vi "外观 2.vi"(0 "Data In":T8 caption="数据输入" {"数值" format="%04x"}, 2 "Display State In":T6 caption="显示状态输入", 3 "Container State":T7 caption="容器状态") -> (6 "Data Out":T8 caption="数据输出" {"数值" format="%04x"}, 7 "Display State Out":T6 caption="显示状态输出", 8 "Action":T5 caption="动作")   [LabVIEW 2016, in "CODMn调试控件V3.xctl"]
uses:
  <vilib>/_xctls/Container State.ctl
  <vilib>/_xctls/Action.ctl
  <vilib>/_xctls/XControlSupport.lvlib
panel:
  in  "模式":enum32{"测试模式", "流程模式"}(tab)
  in  "外设:":T1
  in  "加热:":bool caption="V2"
  in  "摄氏度":u16
  in  "量:":u16=5000
  in  "注射泵:":T2(radio)
  in  "偏心轮:":u16 caption="mL"
  in  "进样:":enum32{"未选择", "水样", "纯水", "标液", "零点", "加标回收"}(radio)
  in  "柱塞泵体积/等待时间":u16=5000
  in  "功能选择":enum32{"等待", "复位", "注入", "注出"}(radio)=enum."注入"
  out "选项卡控件":enum32{"选项卡 1", "选项卡 2"}(tab)
  in  "阀口选择":T3(radio)
  in  "其他":enum32{"未选择", "更新A值", "更新B值", "反滴定"}(radio)
  in  "反应杯温度控制:":u16
  in  "偏心轮抽取液体次数:":u16
  in  "外设":T4
  out "字符串":string="柱塞泵体积μL"
  # "uL"
  # "℃"
  # "次(0代表不动作)"
  # "℃(0代表不控温)"
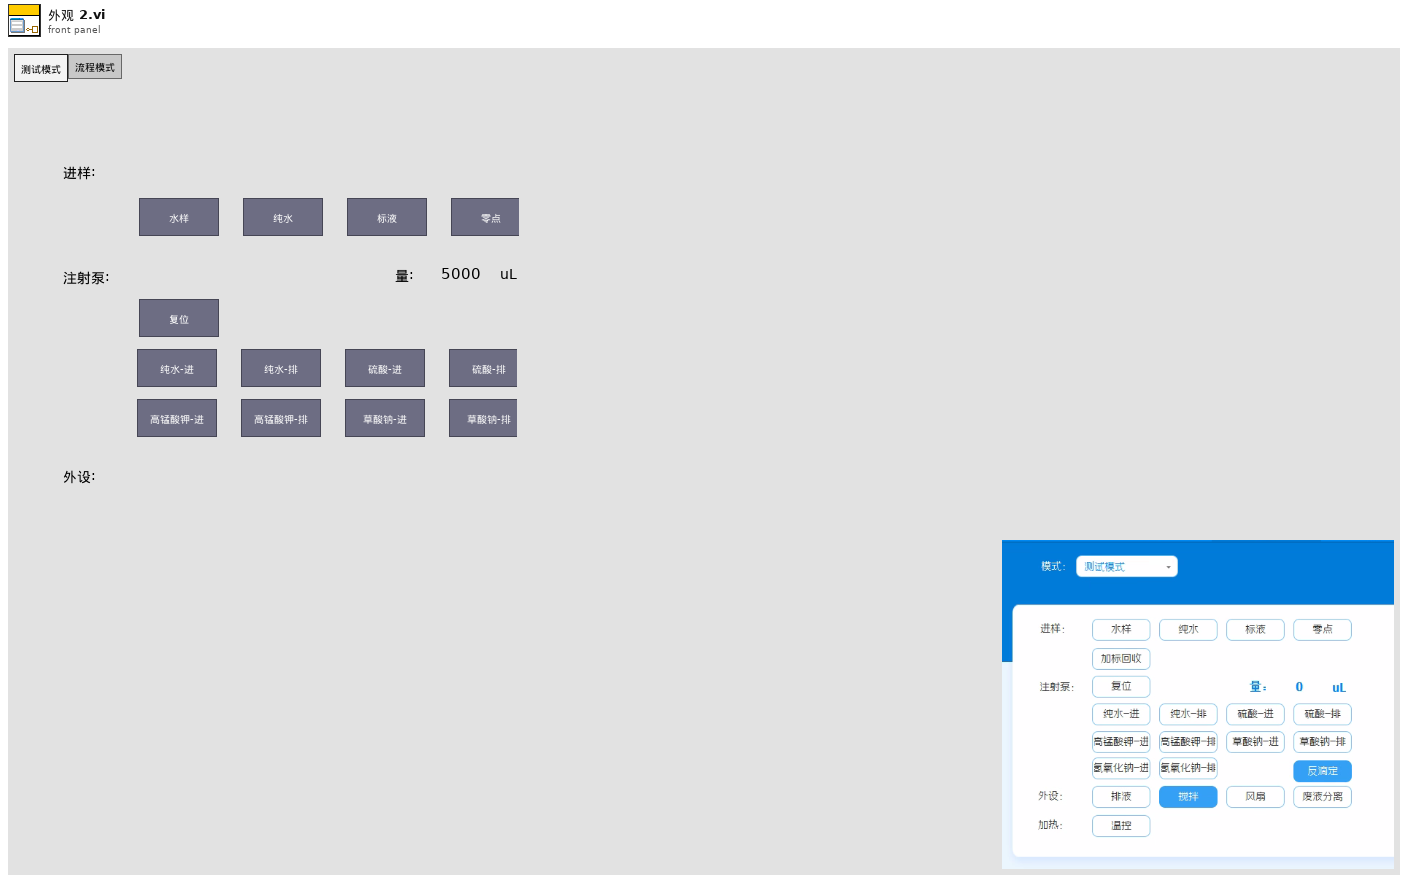
[diagram p1: front panel]
types:
  T1 = cluster{"排液":bool, "搅拌":bool, "风扇":bool, "废液分离":bool}
  T2 = enum32{"未选择", "纯水-进", "纯水-排", "硫酸-进", "硫酸-排", "复位", "高锰酸钾-进", "高锰酸钾-排", "草酸钠-进", "草酸钠-排", "氢氧化钠-进", "氢氧化钠-排", "反滴定"}
  T3 = enum32{"未选择", "V1", "V2", "V3", "V4", "V5", "V6", "V7", "V8", "V9", "V10", "V11", "V12"}
  T4 = cluster{"排液阀":bool, "搅拌":bool, "冷凝风扇":bool, "废液分离阀":bool, "电磁阀1":bool, "电磁阀2":bool, "电磁阀3":bool, "电磁阀4":bool}
  T5 = typedef "XControlSupport.lvlib/Action.ctl" = cluster{"Data Changed?":bool, "State Changed?":bool, "Action Name":string}
  T6 = typedef "CODMn调试控件V3.xctl/状态 2.ctl" = cluster{"Numeric":dbl}
  T7 = typedef "XControlSupport.lvlib/Container State.ctl" = cluster{"Indicator?":bool, "Run Mode?":bool, " Refnum":refnum<vi>}
  T8 = typedef "CODMn调试控件V3.xctl/数据 2.ctl" = cluster{"数值":u16[], "模式":enum32{"测试模式", "流程模式"}}
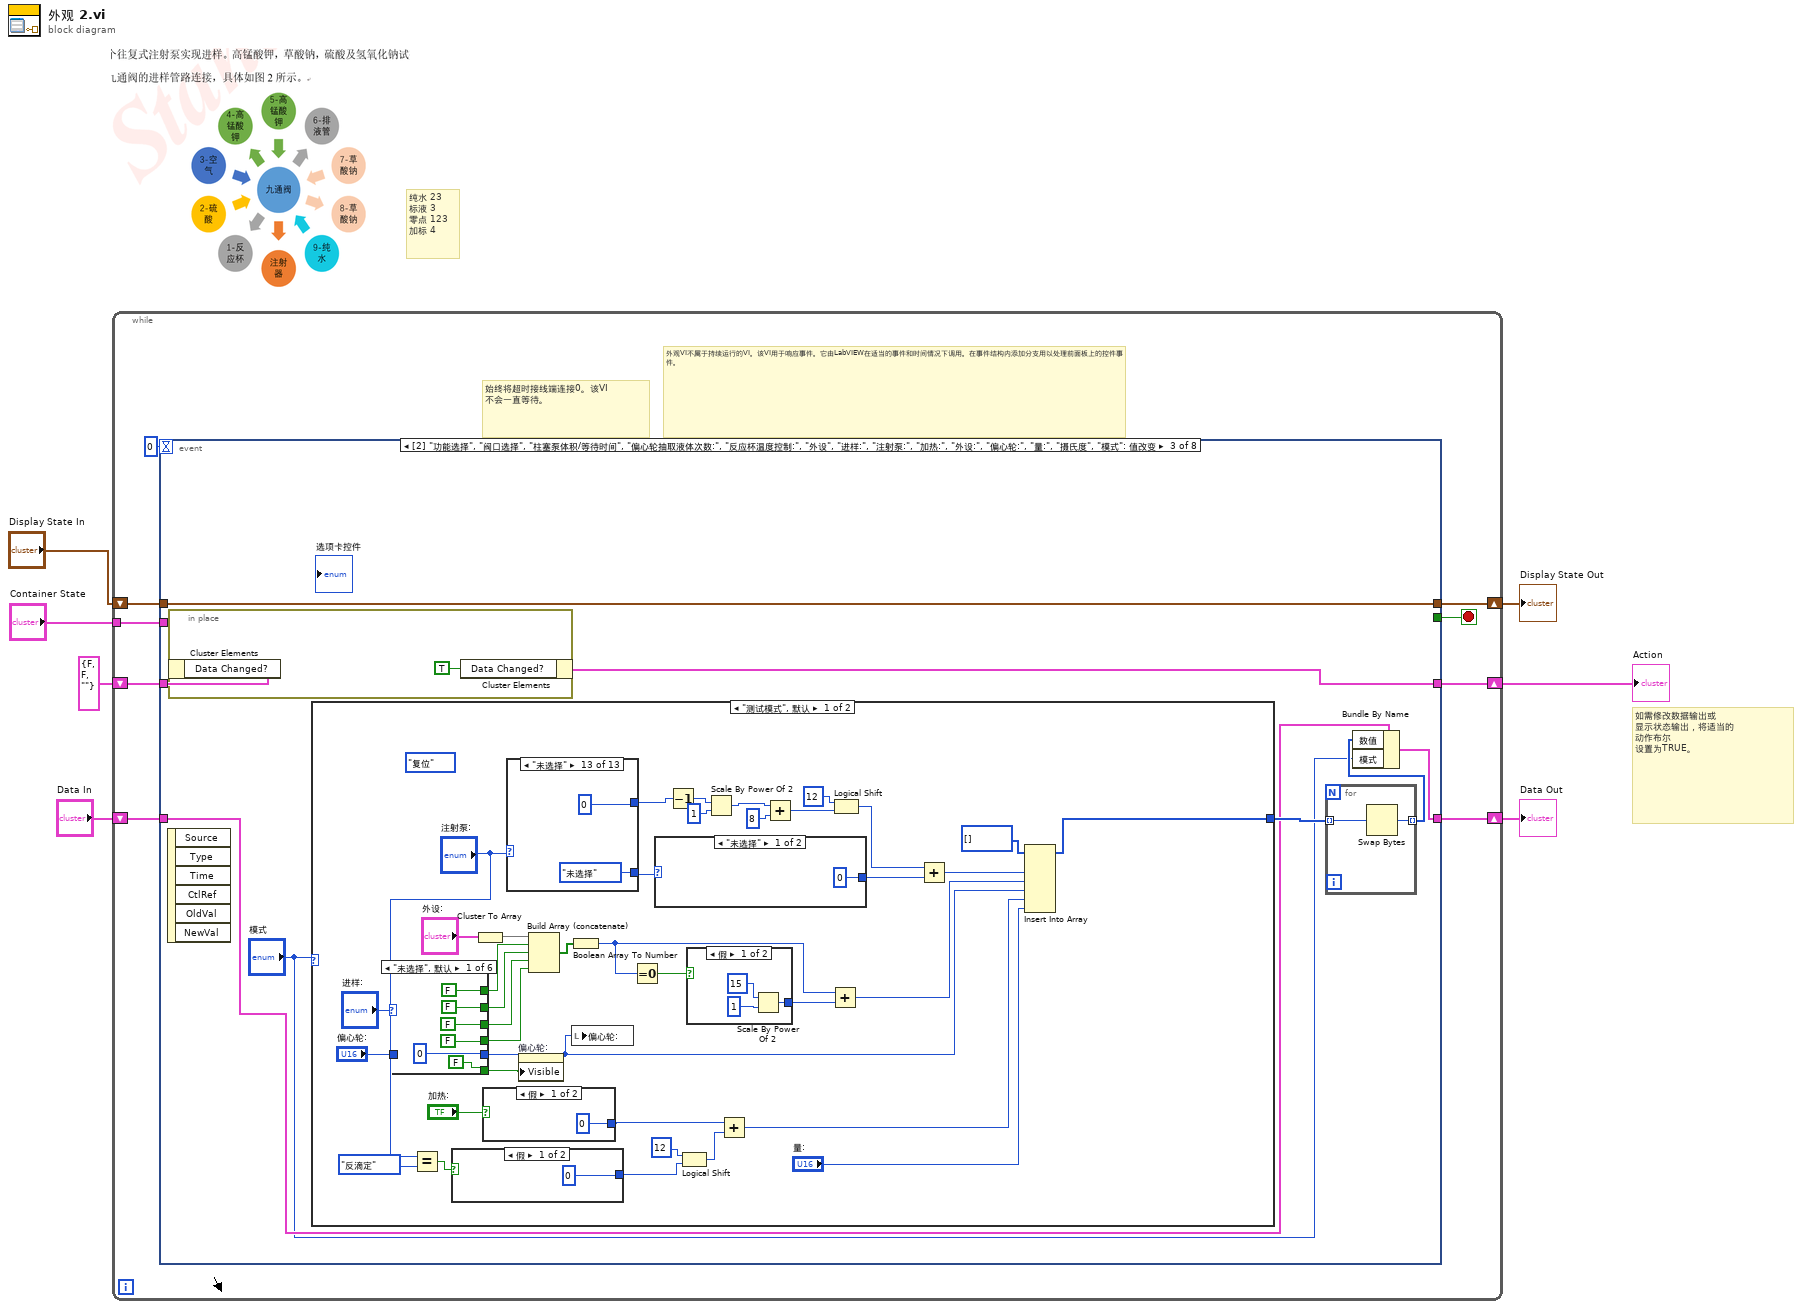
[diagram p0: block diagram]
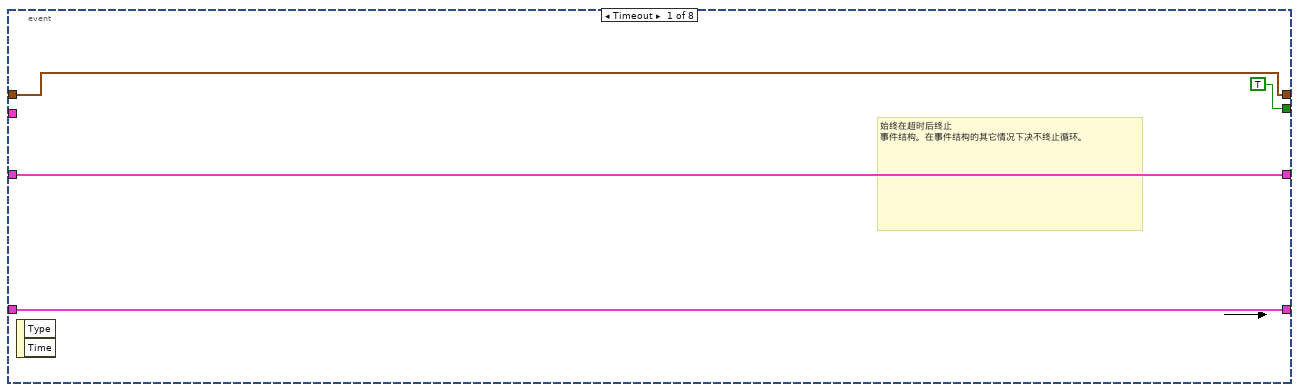
[diagram p2: hidden frame]
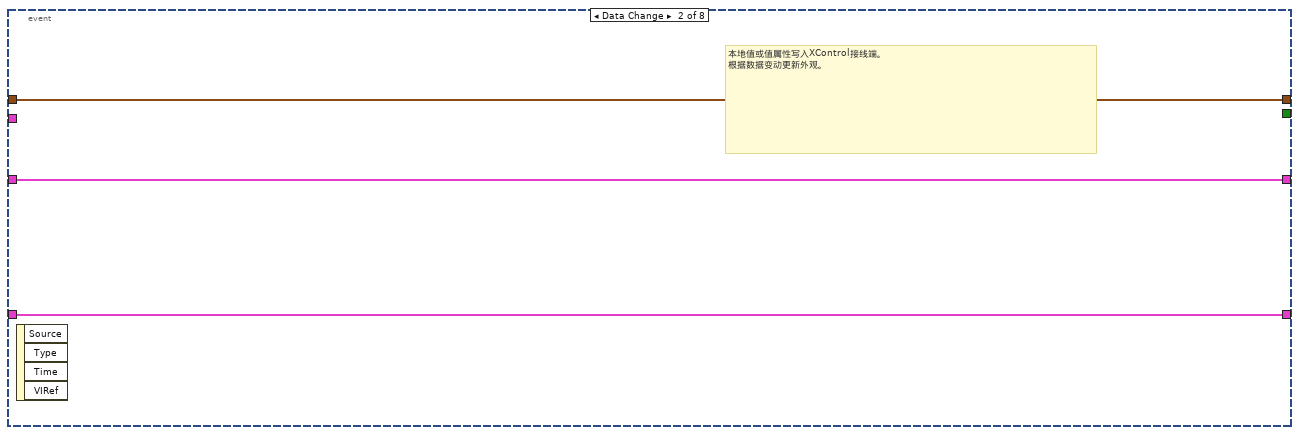
[diagram p3: hidden frame]
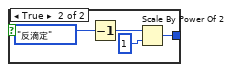
[diagram p4: hidden frame]
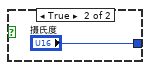
[diagram p5: hidden frame]
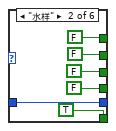
[diagram p6: hidden frame]
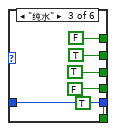
[diagram p7: hidden frame]
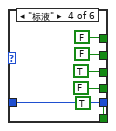
[diagram p8: hidden frame]
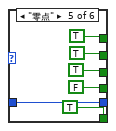
[diagram p9: hidden frame]
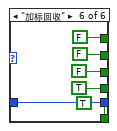
[diagram p10: hidden frame]
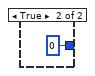
[diagram p11: hidden frame]
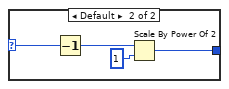
[diagram p12: hidden frame]
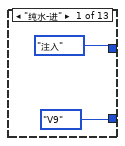
[diagram p13: hidden frame]
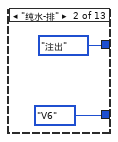
[diagram p14: hidden frame]
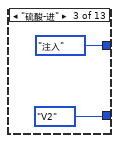
[diagram p15: hidden frame]
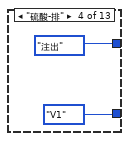
[diagram p16: hidden frame]
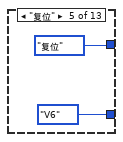
[diagram p17: hidden frame]
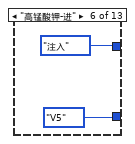
[diagram p18: hidden frame]
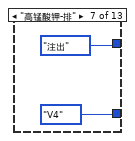
[diagram p19: hidden frame]
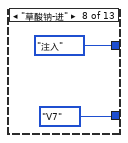
[diagram p20: hidden frame]
diagram:
  # "纯水 23\n标液 3\n零点 123\n加标 4"
  # "如需修改数据输出或\n显示状态输出，将适当的\n动作布尔\n设置为TRUE。"
  n1 = while {
    shift-right: [w15] -> w4
    shift-left: "Display State In" -> [w16]
    tunnel: "Container State" -> [w12]
    shift-right: [w10] -> w7
    shift-left: "Data In" -> [w11]
    shift-right: [w8] -> w2
    shift-left: T5 {"Data Changed?"=FALSE, "State Changed?"=FALSE, "Action Name"=""} ("Action") -> [w9]
    stop <- w14 stop-if-true
    # "外观VI不属于持续运行的VI。该VI用于响应事件。它由LabVIEW在适当的事件和时间情况下调用。在事件结构内添加分支用以处理前面板上的控件事件。"
    # "始终将超时接线端连接0。该VI\n不会一直等待。"
    n2 = event shown="[2] \"功能选择\", \"阀口选择\", \"柱塞泵体积/等待时间\", \"偏心轮抽取液体次数:\", \"反应杯温度控制:\", \"外设\", \"进样:\", \"注射泵:\", \"加热:\", \"外设:\", \"偏心轮:\", \"量:\", \"摄氏度\", \"模式\": 值改变" {
      selector: _ -> [_ _ _ _ _ _ _ _]
      dyn-events: _ -> [_ _ _ _ _ _ _ _]
      timeout: 0 -> [_ _ _ _ _ _ _ _]
      tunnel: w16 -> [w18 w22 w31 w209 w220 w223 w226 w230]
      tunnel: [w18 w22 w31 w209 w220 w223 w226 w230] -> w15
      tunnel: [TRUE _ _ _ _ _ _ _] -> w14
      tunnel: w12 -> [_ _ _ _ _ _ w227 w231]
      tunnel: w11 -> [w17 w23 w27 w208 w219 w222 w225 w229]
      tunnel: [w17 w23 w24 w208 w219 w222 w225 w229] -> w10
      tunnel: [w19 w21 w29 w207 w218 w221 w224 w228] -> w8
      tunnel: w9 -> [w19 w21 w30 w207 w218 w221 w224 w228]
      event Timeout {
        # "始终在超时后终止\n事件结构。在事件结构的其它情况下决不终止循环。"
        n3 = event-data() -> ()  [unwired: 1 in, 2 out]
      }
      event Data Change {
        # "本地值或值属性写入XControl接线端。\n根据数据变动更新外观。"
        n4 = event-data() -> ()  [unwired: 1 in, 4 out]
      }
      event "功能选择", "阀口选择", "柱塞泵体积/等待时间", "偏心轮抽取液体次数:", "反应杯温度控制:", "外设", "进样:", "注射泵:", "加热:", "外设:", "偏心轮:", "量:", "摄氏度", "模式": Value Change {
        n5 = event-data() -> ()  [unwired: 1 in, 6 out]
        n6 = in-place {
          n7 = in-place-cluster #1(w30) -> ()  [unwired: 1 out]
          n8 = in-place-cluster #1("Data Changed?"=TRUE) -> (w29:T5)
        }
        n9 = case shown="\"测试模式\", 默认" "模式" {
          tunnel: [w42 w154] -> w28
          frame "测试模式", Default {
            (unwired) enum32{"等待", "复位", "注入", "注出"}."复位" ("功能选择")
            n10 = case shown="\"未选择\", 默认" "进样:" {
              tunnel: [FALSE FALSE FALSE FALSE TRUE FALSE] -> w59
              tunnel: [FALSE FALSE TRUE FALSE TRUE FALSE] -> w58
              tunnel: [FALSE FALSE TRUE TRUE TRUE FALSE] -> w57
              tunnel: [FALSE FALSE FALSE FALSE FALSE TRUE] -> w56
              tunnel: "偏心轮:" -> [_ w84 w90 w96 w102 w108]
              tunnel: [u16 0 ("偏心轮:") w84 w90 w96 w102 w108] -> w39
              tunnel: [FALSE TRUE TRUE TRUE TRUE TRUE] -> w38
              frame "未选择", Default {
              }
              frame "水样" {
              }
              frame "纯水" {
              }
              frame "标液" {
              }
              frame "零点" {
              }
              frame "加标回收" {
              }
            }
            n11 = Equal?(x="注射泵:", y=T2."反滴定" ("注射泵:")) -> (x = y?=w45:bool)
            n12 = case shown="假" w45 {
              tunnel: [i16 0 w71] -> w44
              frame False {
              }
              frame True {
                n13 = Decrement(x=enum32{"未选择", "更新A值", "更新B值", "反滴定"}."反滴定" ("其他")) -> (x-1=w72:enum32{"未选择", "更新A值", "更新B值", "反滴定"})
                n14 = Scale By Power Of 2(n=w72, x=i16 1 ("y")) -> (x*2^n=w71:i16)
              }
            }
            n15 = Cluster To Array(cluster="外设:") -> (array=w61:bool[])
            n16 = case shown="假" "加热:" {
              tunnel: [u16 0 ("摄氏度") "摄氏度"] -> w48
              frame False {
              }
              frame True {
              }
            }
            n17 = case shown="\"未选择\"" "注射泵:" {
              tunnel: [enum32{"等待", "复位", "注入", "注出"}."注入" ("功能选择") enum32{"等待", "复位", "注入", "注出"}."注出" ("功能选择") enum32{"等待", "复位", "注入", "注出"}."注入" ("功能选择") enum32{"等待", "复位", "注入", "注出"}."注出" ("功能选择") enum32{"等待", "复位", "注入", "注出"}."复位" ("功能选择") enum32{"等待", "复位", "注入", "注出"}."注入" ("功能选择") enum32{"等待", "复位", "注入", "注出"}."注出" ("功能选择") enum32{"等待", "复位", "注入", "注出"}."注入" ("功能选择") enum32{"等待", "复位", "注入", "注出"}."注出" ("功能选择") enum32{"等待", "复位", "注入", "注出"}."注入" ("功能选择") enum32{"等待", "复位", "注入", "注出"}."注出" ("功能选择") 0 0] -> w41
              tunnel: [T3."V9" ("阀口选择") T3."V6" ("阀口选择") T3."V2" ("阀口选择") T3."V1" ("阀口选择") T3."V6" ("阀口选择") T3."V5" ("阀口选择") T3."V4" ("阀口选择") T3."V7" ("阀口选择") T3."V8" ("阀口选择") T3."V3" ("阀口选择") T3."V1" ("阀口选择") T3."未选择" ("阀口选择") T3."未选择" ("阀口选择")] -> w67
              frame "纯水-进" {
              }
              frame "纯水-排" {
              }
              frame "硫酸-进" {
              }
              frame "硫酸-排" {
              }
              frame "复位" {
              }
              frame "高锰酸钾-进" {
              }
              frame "高锰酸钾-排" {
              }
              frame "草酸钠-进" {
              }
              frame "草酸钠-排" {
              }
              frame "氢氧化钠-进" {
              }
              frame "氢氧化钠-排" {
              }
              frame "反滴定" {
              }
              frame "未选择" {
              }
            }
            n18 = property on="偏心轮:" class="DigNum (严格)"("Visible"=w38) -> ()  [unwired: 2 in, 2 out]
            n19 = Build Array (concatenate)(w61, w59, w58, w57, w56) -> (w55:bool[])
            n20 = Boolean Array To Number ("布尔数组至数值转换")(Boolean array=w55) -> (number=w64:u16)
            n21 = local write "偏心轮:"(w39) -> ()
            n22 = Equal To 0?(x=w64) -> (x = 0?=w63:bool)
            n23 = case shown="\"未选择\"" w67 {
              selector: w67 -> [_ w119]
              tunnel: [i16 0 ("y") w121] -> w69
              frame "未选择" {
              }
              frame Default {
                n24 = Decrement(x=w119) -> (x-1=w120:T3)
                n25 = Scale By Power Of 2(n=w120, x=i16 1 ("y")) -> (x*2^n=w121:i16)
              }
            }
            n26 = Decrement(x=w41) -> (x-1=w32:u32)
            n27 = Logical Shift(y=i16 12, x=w44) -> (x << y=w49:i16)
            n28 = case shown="假" w63 {
              tunnel: [w113 u16 0] -> w65
              frame False {
                n29 = Scale By Power Of 2(n=i16 15, x=u16 1 ("y")) -> (x*2^n=w113:u16)
              }
              frame True {
              }
            }
            n30 = Scale By Power Of 2(n=w32, x=i16 1 ("y")) -> (x*2^n=w35:i16)
            n31 = Add(x=w48, y=w49) -> (x+y=w43:u16)
            n32 = Add(x=w35, y=i16 8) -> (x+y=w36:i16)
            n33 = Add(x=w64, y=w65) -> (x+y=w53:u16)
            n34 = Logical Shift(y=i16 12, x=w36) -> (x << y=w68:i16)
            n35 = Add(x=w68, y=w69) -> (x+y=w54:i16)
            n36 = Insert Into Array(array=u16[] [] ("数组"), new element #1=w54, new element #2=w53, new element #3=w39, new element #4=w43, new element #5="量:") -> (w42:u16[])  [unwired: 1 in]
          }
          frame "流程模式" {
            n37 = case shown="默认" "功能选择" {
              selector: "功能选择" -> [_ w188]
              tunnel: [enum32{"选项卡 1", "选项卡 2"}."选项卡 2" ("选项卡控件") enum32{"选项卡 1", "选项卡 2"}."选项卡 1" ("选项卡控件")] -> w160
              tunnel: [w171 u16 0] -> w153
              tunnel: [i16 0 ("y") w189] -> w148
              frame "等待" {
                n38 = Cluster To Array(cluster="外设") -> (array=w172:bool[])
                n39 = Boolean Array To Number ("布尔数组至数值转换")(Boolean array=w172) -> (number=w175:u16)
                n40 = Equal To 0?(x=w175) -> (x = 0?=w174:bool)
                n41 = case shown="假" w174 {
                  tunnel: [w178 u16 0] -> w176
                  frame False {
                    n42 = Scale By Power Of 2(n=i16 15, x=u16 1 ("y")) -> (x*2^n=w178:u16)
                  }
                  frame True {
                  }
                }
                n43 = Add(x=w175, y=w176) -> (x+y=w171:u16)
              }
              frame Default {
                n44 = Decrement(x=w188) -> (x-1=w182:enum32{"等待", "复位", "注入", "注出"})
                n45 = case shown="默认" "阀口选择" {
                  selector: "阀口选择" -> [_ w197]
                  tunnel: [i16 0 ("y") w199] -> w190
                  frame "未选择" {
                  }
                  frame Default {
                    n46 = Decrement(x=w197) -> (x-1=w198:T3)
                    n47 = Scale By Power Of 2(n=w198, x=i16 1 ("y")) -> (x*2^n=w199:i16)
                  }
                }
                n48 = Scale By Power Of 2(n=w182, x=i16 1 ("y")) -> (x*2^n=w185:i16)
                n49 = Add(x=w185, y=i16 8) -> (x+y=w184:i16)
                n50 = Logical Shift(y=i16 12, x=w184) -> (x << y=w191:i16)
                n51 = Add(x=w191, y=w190) -> (x+y=w189:i16)
              }
            }
            n52 = case shown="\"更新A值\", 默认" "其他" {
              tunnel: "其他" -> [_ w166]
              tunnel: [i16 0 w165] -> w151
              frame "未选择" {
              }
              frame "更新A值", Default {
                n53 = Decrement(x=w166) -> (x-1=w168:enum32{"未选择", "更新A值", "更新B值", "反滴定"})
                n54 = Scale By Power Of 2(n=w168, x=i16 1 ("y")) -> (x*2^n=w165:i16)
              }
            }
            n55 = Logical Shift(y=i16 12, x=w151) -> (x << y=w150:i16)
            n56 = feedback #2() -> (w162:enum32{"选项卡 1", "选项卡 2"})  [unwired: 1 in]
            n57 = feedback-in #2(w160) -> ()
            n58 = Add(x="反应杯温度控制:", y=w150) -> (x+y=w155:u16)
            n59 = Not Equal?(x=w160, y=w162) -> (x != y?=w161:bool)
            n60 = case shown="真" w161 {
              tunnel: w160 -> [_ w169]
              frame False {
              }
              frame True {
                n61 = property on="选项卡控件" class="TabCtl (严格)"("Val(Sgnl)"=w169) -> ()  [unwired: 2 in, 2 out]
              }
            }
            n62 = Insert Into Array(array=u16[] [] ("数组"), new element #1=w148, new element #2=w153, new element #3="偏心轮抽取液体次数:", new element #4=w155, new element #5="柱塞泵体积/等待时间") -> (w154:u16[])  [unwired: 1 in]
          }
        }
        n63 = for {
          tunnel: w28 -> [w201] mode=indexing
          tunnel: [w200] -> w26 mode=indexing
          n64 = Swap Bytes(anything=w201) -> (byte swapped=w200:u16)
        }
        n65 = Bundle By Name(cluster=w27, "数值"=w26, "模式"="模式") -> (w24:T8)
      }
      event "选项卡控件": Value Change {
        n66 = event-data() -> ("NewVal"=w206:enum32{"选项卡 1", "选项卡 2"})  [unwired: 1 in, 5 out]
        n67 = case shown="\"选项卡 1\", 默认" w206 {
          tunnel: [i16 5000 ("数值") i16 60 ("数值")] -> w205
          tunnel: ["柱塞泵体积μL" ("字符串") "等待时间秒" ("字符串")] -> w203
          frame "选项卡 1", Default {
          }
          frame "选项卡 2" {
          }
        }
        "字符串" <- w203
        n68 = local write "阀口选择"(T3."未选择" ("阀口选择")) -> ()
        n69 = local write "柱塞泵体积/等待时间"(w205) -> ()
      }
      event "柱塞泵体积/等待时间", "偏心轮抽取液体次数:", "反应杯温度控制:", "偏心轮:", "量:", "摄氏度": Mouse Down {
        n70 = event-data() -> ("CtlRef"=w217:refnum<vi>)  [unwired: 1 in, 7 out]
        n71 = property class="DigNum (严格)"(reference=w217) -> (reference out=w216:refnum<vi>, "Value"=w215:u16)  [unwired: 1 in, 1 out]
        n72 = call "数字键盘.vi"("OldNumber"=w215) -> ("NewNumber"=w214:sgl)
        n73 = property class="DigNum (严格)"(reference=w216, "Val(Sgnl)"=w214) -> ()  [unwired: 1 in, 2 out]
      }
      event Display State Change {
        # "拖放该XControl的新实例、复制、撤消操作或者在XControl内执行自定义属性或方法均可改变显示状态。更新相应外观。"
        n74 = event-data() -> ()  [unwired: 1 in, 4 out]
      }
      event Direction Change {
        # "XControl的方向由输入控件转换为显示控件，反之亦然。更新相应外观。"
        n75 = event-data() -> ()  [unwired: 1 in, 4 out]
        n76 = Unbundle By Name(w227) -> ()  [unwired: 1 out]
      }
      event Exec State Change {
        # "包含该XControl的VI已从编辑模式切换至运行模式，反之亦然。\n相应的更新外观。"
        # "分别处理编辑模式和\n运行模式"
        n77 = event-data() -> ()  [unwired: 1 in, 4 out]
        n78 = Unbundle By Name(w231) -> ()  [unwired: 1 out]
      }
    }
  }
  "Display State Out" <- w4
  "Data Out" <- w7
  "Action" <- w2
